vi "Export plot data to Clipboard.vi"(3 "VI caller":refnum<vi>, 4 "List Plots":string[](array[string]), 5 "Graph reference":refnum<vi>) -> (2 "Ready?":bool)   [LabVIEW 2022 SP3]
panel:
  in  "Plot":string(combo)
  in  "Export":bool
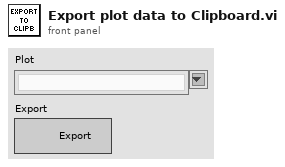
[diagram p1: front panel]
types:
  T1 = enum32{"Invalid", "Standard", "Closed", "Hidden", "Minimized", "Maximized"}
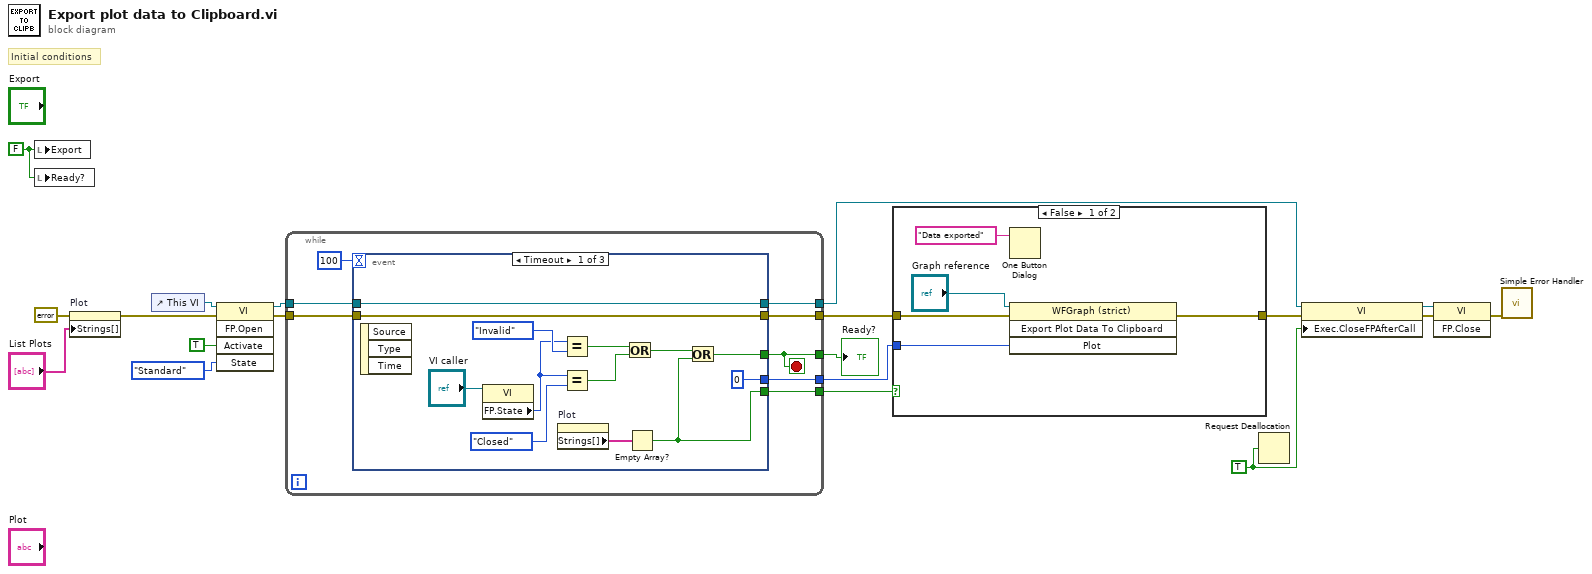
[diagram p0: block diagram]
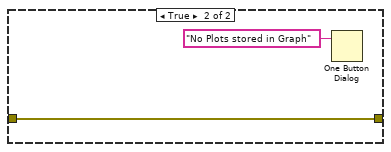
[diagram p2: hidden frame]
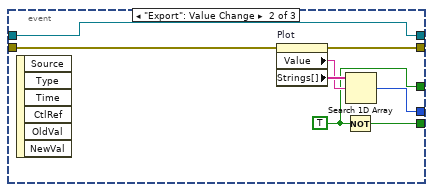
[diagram p3: hidden frame]
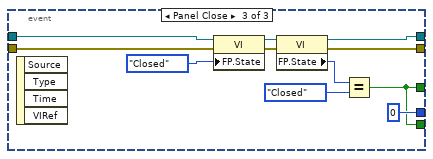
[diagram p4: hidden frame]
diagram:
  w1 = TRUE ("Activate?")
  w10 = FALSE
  # "Initial conditions"
  n1 = local write "Export"(w10) -> ()
  n2 = local write "Ready?"(w10) -> ()
  n3 = property on="Plot" class="CmbBox"(error in=errorcluster {"status"=FALSE, "code"=0, "source"=""} ("error in (no error)"), "Strings[]"="List Plots") -> (error out=w5:errorcluster)  [unwired: 1 in, 1 out]
  n4 = control-ref of="This VI"() -> (w8:refnum<vi>)
  n5 = invoke on="Invoke Node" class="VI" method="FP.Open"(reference=w8, error in=w5, "Activate"=TRUE ("Activate?"), "State"=T1."Standard") -> (reference out=w16:refnum<vi>, error out=w17:errorcluster)  [unwired: 1 in, 3 out]
  n6 = while {
    tunnel: [w22] -> w19
    tunnel: w17 -> [w26]
    tunnel: w16 -> [w24]
    tunnel: [w23] -> w14
    tunnel: [w25] -> w13
    tunnel: [w27] -> w9
    tunnel: [w20] -> w3
    stop <- w22 stop-if-true
    n7 = event shown="[0] Timeout" {
      selector: _ -> [_ _ _]
      dyn-events: _ -> [_ _ _]
      timeout: 100 -> [_ _ _]
      tunnel: [w29 w42 w49] -> w22
      tunnel: [0 ("index of element") w46 0 ("index of element")] -> w27
      tunnel: w26 -> [w39 w44 w55]
      tunnel: [w39 w43 w53] -> w25
      tunnel: w24 -> [w38 w45 w52]
      tunnel: [w38 w45 w51] -> w23
      tunnel: [w28 w41 w49] -> w20
      event Timeout {
        n8 = event-data() -> ()  [unwired: 1 in, 3 out]
        n9 = property class="VI"(reference="VI caller") -> ("FP.State"=w35:T1)  [unwired: 1 in, 2 out]
        n10 = property on="Plot" class="CmbBox"() -> ("Strings[]"=w31:string[])  [unwired: 2 in, 2 out]
        n11 = Equal?(x=w35, y=T1."Invalid" ("Front Panel Window:State")) -> (x = y?=w32:bool)
        n12 = Equal?(x=w35, y=T1."Closed" ("Front Panel Window:State")) -> (x = y?=w33:bool)
        n13 = Or(x=w32, y=w33) -> (x .or. y?=w30:bool)
        n14 = Empty Array?(array=w31) -> (empty?=w28:bool)
        n15 = Or(x=w30, y=w28) -> (x .or. y?=w29:bool)
      }
      event "Export": Value Change {
        w42 = TRUE
        n16 = event-data() -> ()  [unwired: 1 in, 6 out]
        n17 = property on="Plot" class="CmbBox"(error in=w44) -> (error out=w43:errorcluster, "Value"=w47:string, "Strings[]"=w48:string[])  [unwired: 1 in, 1 out]
        n18 = Not(x=w42) -> (.not. x?=w41:bool)
        n19 = Search 1D Array(1D array=w48, element=w47) -> (index of element=w46:i32)  [unwired: 1 in]
      }
      event Panel Close {
        n20 = event-data() -> ()  [unwired: 1 in, 4 out]
        n21 = property class="VI"(reference=w52, error in=w55, "FP.State"=T1."Closed" ("Front Panel Window:State")) -> (reference out=w56:refnum<vi>, error out=w54:errorcluster)
        n22 = property class="VI"(reference=w56, error in=w54) -> (reference out=w51:refnum<vi>, error out=w53:errorcluster, "FP.State"=w59:T1)
        n23 = Equal?(x=w59, y=T1."Closed" ("Front Panel Window:State")) -> (x = y?=w49:bool)
      }
    }
  }
  "Ready?" <- w19
  n24 = case shown="False" w3 {
    tunnel: w13 -> [w64 w66]
    tunnel: w9 -> [w63 _]
    tunnel: [w61 w66] -> w7
    frame False {
      n25 = One Button Dialog(message="Data exported") -> ()  [unwired: 1 in, 1 out]
      n26 = invoke on="Invoke Node" class="WFGraph (strict)" method="Export Plot Data To Clipboard"(reference="Graph reference", error in=w64, "Plot"=w63) -> (error out=w61:errorcluster)  [unwired: 1 in, 3 out]
    }
    frame True {
      n27 = One Button Dialog(message="No Plots stored in Graph") -> ()  [unwired: 1 in, 1 out]
    }
  }
  n28 = Request Deallocation(w1) -> ()
  n29 = property class="VI"(reference=w14, error in=w7, "Exec.CloseFPAfterCall"=w1) -> (reference out=w12:refnum<vi>, error out=w11:errorcluster)
  n30 = invoke class="VI" method="FP.Close"(reference=w12, error in=w11) -> (error out=w2:errorcluster)  [unwired: 1 in, 2 out]
  n31 = call <vilib>:"Simple Error Handler.vi"("error in (no error)"=w2) -> ()  [unwired: 4 in, 5 out]
